vi "数据格式转化.vi"() -> ()   [LabVIEW 2020]
uses:
  <vilib>/drjdpowell/SQLite Library/SQL Connection/Connection.lvclass
  <vilib>/drjdpowell/SQLite Library/SQLite.lvlib
  <vilib>/drjdpowell/SQLite Library/SQL Connection/Execute SQL (No results).vi
  <vilib>/drjdpowell/SQLite Library/SQL Connection/Open (path).vi
  <vilib>/JDP Science/JDP Science Common Utilities/Base64/Base64 Support.lvlib
panel:
  out "进度":i32(slide)
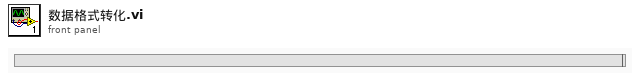
[diagram p1: front panel]
types:
  T1 = enum16{"open", "open or create", "create or replace", "create", "open (read-only)"}
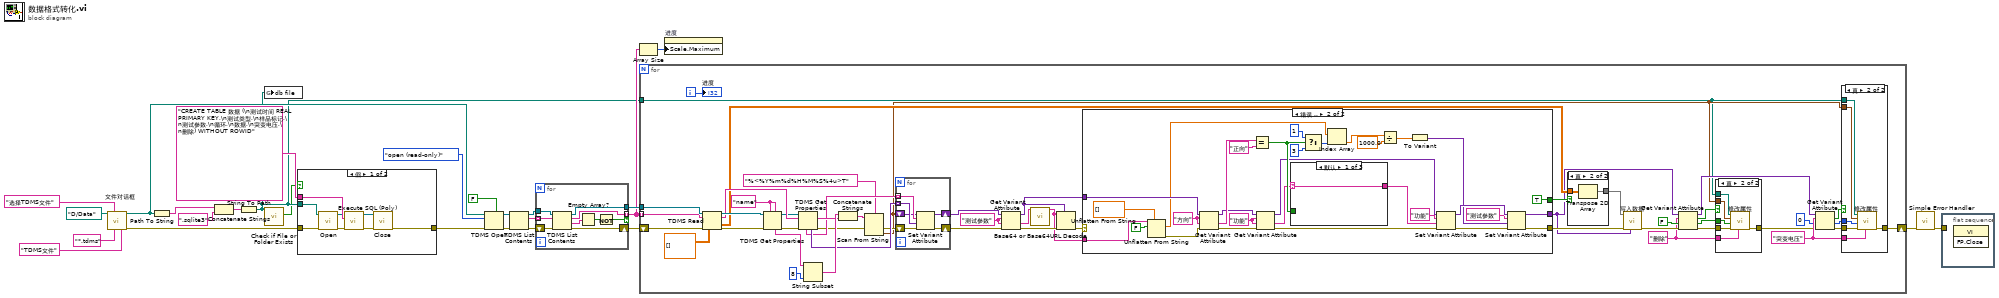
[diagram p0: block diagram]
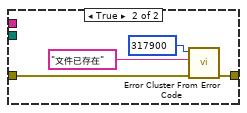
[diagram p2: hidden frame]
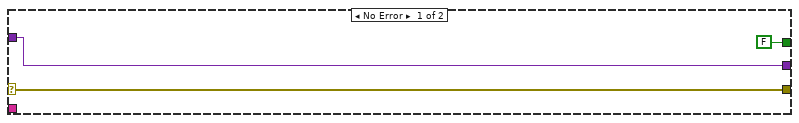
[diagram p5: hidden frame]
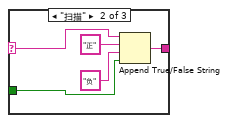
[diagram p6: hidden frame]
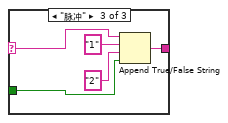
[diagram p7: hidden frame]
diagram:
  n1 = call "文件对话框"("start path"=path "D:/Data", "prompt"="选择TDMS文件", "pattern (all files)"="*.tdms", "pattern label"="TDMS文件") -> ("selected path"=w13:path, "error out"=w8:errorcluster)  [unwired: 8 in, 2 out]
  n2 = Path To String(path=w13) -> (string=w12:string)
  n3 = Concatenate Strings(w12, ".sqlite3" ("字符串")) -> (w10:string)
  n4 = String To Path(string=w10) -> (path=w2:path)
  n5 = global write "数据库.vi" "db file"(w2) -> ()
  n6 = call <vilib>:"Check if File or Folder Exists.vi"("path"=w2) -> ("file or folder exists?"=w1:bool)  [unwired: 8 in, 2 out]
  n7 = case shown="假" w1 {
    tunnel: "CREATE TABLE 数据 (\n测试时间 REAL PRIMARY KEY,\n测试类型,\n样品标记,\n测试参数,\n循环,\n数据,\n突变电压,\n删除) WITHOUT ROWID" -> [w34 _]
    tunnel: w8 -> [w33 w35]
    tunnel: [w32 w38] -> w7
    tunnel: w2 -> [w27 _]
    frame False {
      n8 = call-poly <vilib>:"Open.vi"("error in (no error)"=w33, "db file"=w27) -> ("error out"=w30:errorcluster, "SQLite Connection"=w31:refnum<class "Connection.lvclass">)  [unwired: 8 in]
      n9 = call-poly <vilib>:"Execute SQL (Poly).vi"("error in (no error)"=w30, "SQL"=w34, "SQLite Connection in"=w31) -> ("error out"=w29:errorcluster, "SQLite Connection"=w28:refnum<class "Connection.lvclass">)  [unwired: 7 in]
      n10 = call-dynamic "Close.vi"("error in (no error)"=w29, "SQLite Connection in"=w28) -> ("error out"=w32:errorcluster)  [unwired: 9 in]
    }
    frame True {
      n11 = call <vilib>:"Error Cluster From Error Code.vi"("error in (no error)"=w35, "error message (\"\")"="文件已存在" ("error message (\"\")"), "error code (0)"=317900) -> ("error out"=w38:errorcluster)  [unwired: 6 in]
    }
  }
  n12 = TDMS Open(5:FALSE ("创建索引文件？(T)"), 8:w7, 10:T1."open (read-only)" ("操作(0:open)"), 11:w13) -> (0:w21:errorcluster, 3:w20:refnum<k34>)  [unwired: 3 in]
  n13 = TDMS List Contents(4:w21, 7:w20) -> (0:w15:errorcluster, 2:w16:string[], 3:w17:refnum<k34>)  [unwired: 1 in, 1 out]
  n14 = for {
    tunnel: w17 -> [w47]
    tunnel: w16 -> [w46] mode=indexing
    tunnel: [w43] -> w19
    tunnel: [w42] -> w5 mode=indexing if=w39
    shift-right: [w41] -> w18
    shift-left: w15 -> [w45]
    n15 = TDMS List Contents(4:w45, 6:w46, 7:w47) -> (0:w41:errorcluster, 1:w44:string[], 2:w42:string, 3:w43:refnum<k34>)
    n16 = Empty Array?(array=w44) -> (empty?=w40:bool)
    n17 = Not(x=w40) -> (.not. x?=w39:bool)
  }
  n18 = Array Size(array=w5) -> (size(s)=w4:i32)
  n19 = for {
    tunnel: w19 -> [w97]
    tunnel: w5 -> [w95] mode=indexing
    shift-right: [w49] -> w6
    shift-left: w18 -> [w94]
    tunnel: w2 -> [w51]
    i -> [w48]
    w56 = "突变电压" ("名称")
    w61 = "删除" ("名称")
    w76 = "name" ("属性名称")
    w84 = "测试参数" ("名称")
    n20 = TDMS Read(0:w97, 5:w95, 11:w94, 12:dbl[][] []) -> (4:w93:refnum<k34>, 6:w92:string, 10:w89:dbl[][], 15:w91:errorcluster)  [unwired: 4 in, 2 out]
    n21 = TDMS Get Properties(5:w76, 7:w76, 8:w91, 11:w93) -> (0:w72:errorcluster, 3:w73:refnum<k34>, 4:w79:string)  [unwired: 2 in, 3 out]
    n22 = TDMS Get Properties(8:w72, 10:w92, 11:w73) -> (0:w71:errorcluster, 2:w80:string, 4:w78:variant[], 6:w77:string[])  [unwired: 3 in, 2 out]
    n23 = String Subset(string=w79, length (rest)=8 ("长度（剩余）")) -> (substring=w81:string)  [unwired: 1 in]
    n24 = Concatenate Strings(w81, w80) -> (w75:string)
    n25 = Scan From String(format string="%<%Y%m%d%H%M%S%4u>T" ("格式字符串"), input string=w75, error in=w71) -> (error out=w70:errorcluster, output 1=w52:timestamp)  [unwired: 2 in, 2 out]
    n26 = for {
      tunnel: w77 -> [w117] mode=indexing
      tunnel: w78 -> [w116] mode=indexing
      shift-right: [w115] -> w66
      shift-left: w52 -> [w114]
      shift-right: [w112] -> w67
      shift-left: w70 -> [w113]
      n27 = Set Variant Attribute(Variant=w114, name=w117, value=w116, error in=w113) -> (Variant out=w115:variant, error out=w112:errorcluster)  [unwired: 1 out]
    }
    n28 = Get Variant Attribute(Variant=w66, name=w84, default value (empty Variant)=w84, error in=w67) -> (duplicate Variant=w88:variant, value=w83:string, error out=w87:errorcluster)  [unwired: 1 out]
    n29 = call <vilib>:"Base64 or Base64URL Decode.vi"("Base64 or Base64URL"=w83) -> ("Decoded"=w86:string)  [unwired: 10 in]
    n30 = Unflatten From String(type=w88, binary string=w86, error in (no error)=w87) -> (error out=w85:errorcluster)  [unwired: 2 in, 2 out]
    n31 = case shown="错误 .." w85 {
      selector: w85 -> [w120 _]
      tunnel: [w120 w132] -> w68
      tunnel: w86 -> [_ w150]
      tunnel: [w118 w128] -> w63
      tunnel: w88 -> [w118 w148]
      tunnel: [FALSE TRUE] -> w90
      frame No Error {
      }
      frame Error {
        w127 = "功能" ("名称")
        w147 = "方向" ("名称")
        n32 = Unflatten From String(type=dbl[] [], binary string=w150, data includes array or string size? (T)=FALSE ("数据中包含数组或字符串大小？(T)")) -> (value=w144:dbl[], error out=w124:errorcluster)  [unwired: 2 in, 1 out]
        n33 = Get Variant Attribute(Variant=w148, name=w147, default value (empty Variant)=w147, error in=w124) -> (duplicate Variant=w122:variant, value=w146:string, error out=w125:errorcluster)  [unwired: 1 out]
        n34 = Equal?(x=w146, y="正向") -> (x = y?=w136:bool)
        n35 = Get Variant Attribute(Variant=w122, name=w127, default value (empty Variant)=w127, error in=w125) -> (duplicate Variant=w121:variant, value=w126:string, error out=w123:errorcluster)  [unwired: 1 out]
        n36 = case shown="默认" w126 {
          selector: w126 -> [w152 w157 w162]
          tunnel: w136 -> [_ w156 w161]
          tunnel: [w152 w153 w158] -> w134
          frame Default {
          }
          frame "扫描" {
            n37 = Append True/False String(1:w156, 2:"负" ("假字符串"), 3:"正" ("真字符串"), 4:w157) -> (0:w153:string)
          }
          frame "脉冲" {
            n38 = Append True/False String(1:w161, 2:"2" ("假字符串"), 3:"1" ("真字符串"), 4:w162) -> (0:w158:string)
          }
        }
        n39 = Select(t=1 ("索引"), s=w136, f=3) -> (s? t:f=w141:i32)
        n40 = Index Array(array=w144, index=w141) -> (element=w138:dbl)
        n41 = Divide(x=w138, y=1000.0) -> (x/y=w139:dbl)
        n42 = To Variant(anything=w139) -> (Variant=w130:variant)
        n43 = Set Variant Attribute(Variant=w121, name="功能" ("名称"), value=w134, error in=w123) -> (Variant out=w131:variant, error out=w133:errorcluster)  [unwired: 1 out]
        n44 = Set Variant Attribute(Variant=w131, name="测试参数" ("名称"), value=w130, error in=w133) -> (Variant out=w128:variant, error out=w132:errorcluster)  [unwired: 1 out]
      }
    }
    n45 = case shown="真" w90 {
      tunnel: w89 -> [w163 w165]
      tunnel: [w163 w164] -> w69
      frame False {
      }
      frame True {
        n46 = Transpose 2D Array(2D array=w165) -> (transposed array=w164:dbl[][])
      }
    }
    n47 = call "写入数据.vi"("数据属性"=w63, "错误输入（无错误）"=w68, "测试数据"=w69) -> ("错误输出"=w65:errorcluster)  [unwired: 8 in]
    n48 = Get Variant Attribute(Variant=w63, name=w61, default value (empty Variant)=FALSE, error in=w65) -> (duplicate Variant=w53:variant, found=w59:bool, value=w60:bool, error out=w64:errorcluster)
    n49 = case shown="真" w59 {
      tunnel: [w105 w111] -> w54
      tunnel: w64 -> [w105 w110]
      tunnel: w52 -> [_ w109]
      tunnel: w51 -> [_ w108]
      tunnel: w61 -> [_ w107]
      tunnel: w60 -> [_ w106]
      frame False {
      }
      frame True {
        n50 = call "修改属性.vi"("属性名称"=w107, "错误输入（无错误）"=w110, "属性值"=w106, "测试时间"=w109, "db file"=w108) -> ("错误输出"=w111:errorcluster)  [unwired: 6 in]
      }
    }
    n51 = Get Variant Attribute(Variant=w53, name=w56, default value (empty Variant)=0, error in=w54) -> (found=w58:bool, value=w57:i32, error out=w55:errorcluster)  [unwired: 1 out]
    n52 = case shown="真" w58 {
      tunnel: [w98 w104] -> w49
      tunnel: w55 -> [w98 w103]
      tunnel: w52 -> [_ w102]
      tunnel: w51 -> [_ w101]
      tunnel: w56 -> [_ w100]
      tunnel: w57 -> [_ w99]
      frame False {
      }
      frame True {
        n53 = call "修改属性.vi"("属性名称"=w100, "错误输入（无错误）"=w103, "属性值"=w99, "测试时间"=w102, "db file"=w101) -> ("错误输出"=w104:errorcluster)  [unwired: 6 in]
      }
    }
    "进度" <- w48
  }
  n54 = property on="进度" class="Slide (严格)"("Scale.Maximum"=w4) -> ()  [unwired: 2 in, 2 out]
  n55 = call <vilib>:"Simple Error Handler.vi"("error in (no error)"=w6) -> ("error out"=w3:errorcluster)  [unwired: 4 in, 4 out]
  n56 = flat-sequence {
    tunnel: w3 -> [_]
    frame #0 {
      n57 = invoke class="VI" method="FP.Close"() -> ()  [unwired: 3 in, 3 out]
    }
  }
